vi "Debug_MessageToString.vi"(11 "TrackerData":T1) -> (3 "Array":string[](array[string]))   [LabVIEW 2017, in "Server.lvlib" / "Message Queue.lvlib"]
doc: "This VI formats the Tracker-Cluster from the TrackerQueue to a 1D-String-Array. The Variant is displayed in its XML-Notation!"
uses:
  Message Queue.lvlib
  Debug_TrackerData.ctl
  MessageCluster.ctl
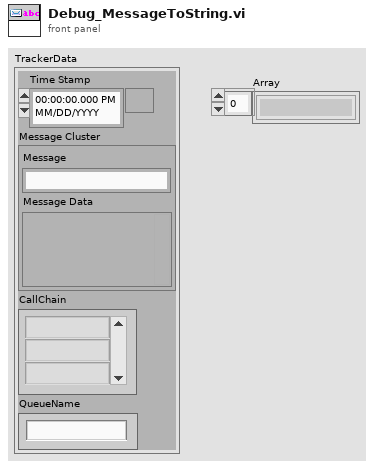
[diagram p1: front panel]
types:
  T1 = typedef "Server.lvlib/Message Queue.lvlib/Debug_TrackerData.ctl" = cluster{"Time Stamp":timestamp, "Message Cluster":T2, "CallChain":string[], "QueueName":string}
  T2 = typedef "Server.lvlib/Message Queue.lvlib/MessageCluster.ctl" = cluster{"Message":string, "Message Data":variant}
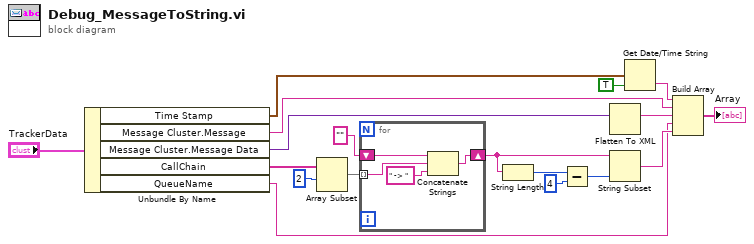
[diagram p0: block diagram]
diagram:
  n1 = Unbundle By Name("TrackerData") -> ("Time Stamp"=w11:timestamp, "Message Cluster.Message"=w6:string, "Message Cluster.Message Data"=w7:variant, "CallChain"=w2:string[], "QueueName"=w9:string)
  n2 = Array Subset(array=w2, index=2) -> (w4:string[])  [unwired: 1 in]
  n3 = for {
    tunnel: w4 -> [w22] mode=indexing
    shift-right: [w20] -> w15
    shift-left: "" -> [w19]
    n4 = Concatenate Strings(w19, w22, " -> " ("string")) -> (w20:string)
  }
  n5 = String Length(string=w15) -> (length=w16:i32)
  n6 = Subtract(x=w16, y=4) -> (x-y=w18:i32)
  n7 = Flatten To XML(anything=w7) -> (xml string=w8:string)
  n8 = String Subset(string=w15, length (rest)=w18) -> (substring=w14:string)  [unwired: 1 in]
  n9 = Get Date/Time String(seconds (now)=w11, want seconds? (F)=TRUE) -> (time string=w13:string)  [unwired: 1 in, 1 out]
  n10 = Build Array(w13, w6, w8, w9, w14) -> (→"Array":string[])
